vi "Actor Core.vi"(8 "error in":cluster{"状态":bool, "代码":i32, "源":string} caption="错误输入", 11 "客户端":refnum<class "客户端.lvclass"> caption="DNL_Beta") -> (0 "error out":cluster{"状态":bool, "代码":i32, "源":string} caption="错误输出", 3 "操作者输出":refnum<class "Actor.lvclass">)   [LabVIEW 2015, in "客户端操作者.lvlib" / "客户端.lvclass"]
doc: "Actor Core.vi包含操作者的主要消息处理循环。操作者通常位于该循环中，在各种消息到达时对消息进行处理。如Do.vi消息返回任何错误，该循环将停止运行，错误代码43将被作为“无错误停止”的标准信号发送给调用方。如需更改上述行为，可在子孙类的Handle Error.vi中对该部分逻辑进行重写。"
uses:
  <vilib>/ActorFramework/Actor/Actor.lvclass
panel:
  out "接收":string
  in  "发送按钮":bool
  in  "发送":string
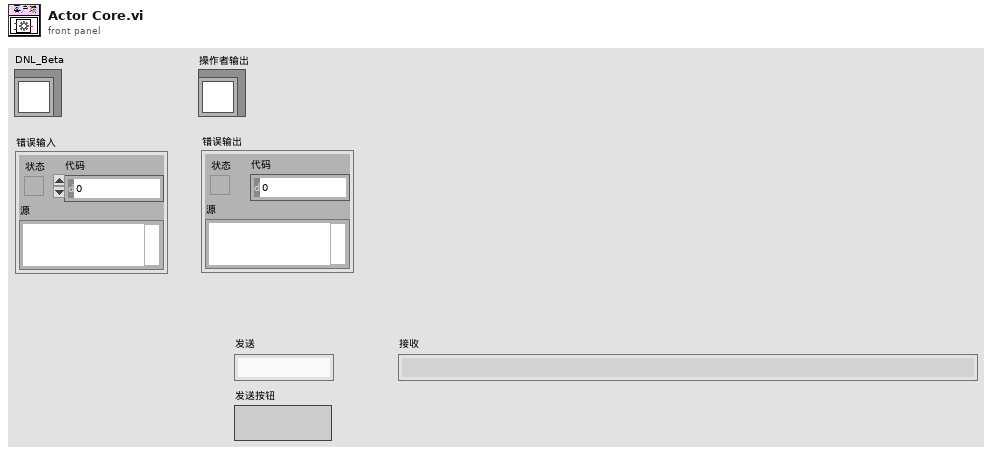
[diagram p1: front panel]
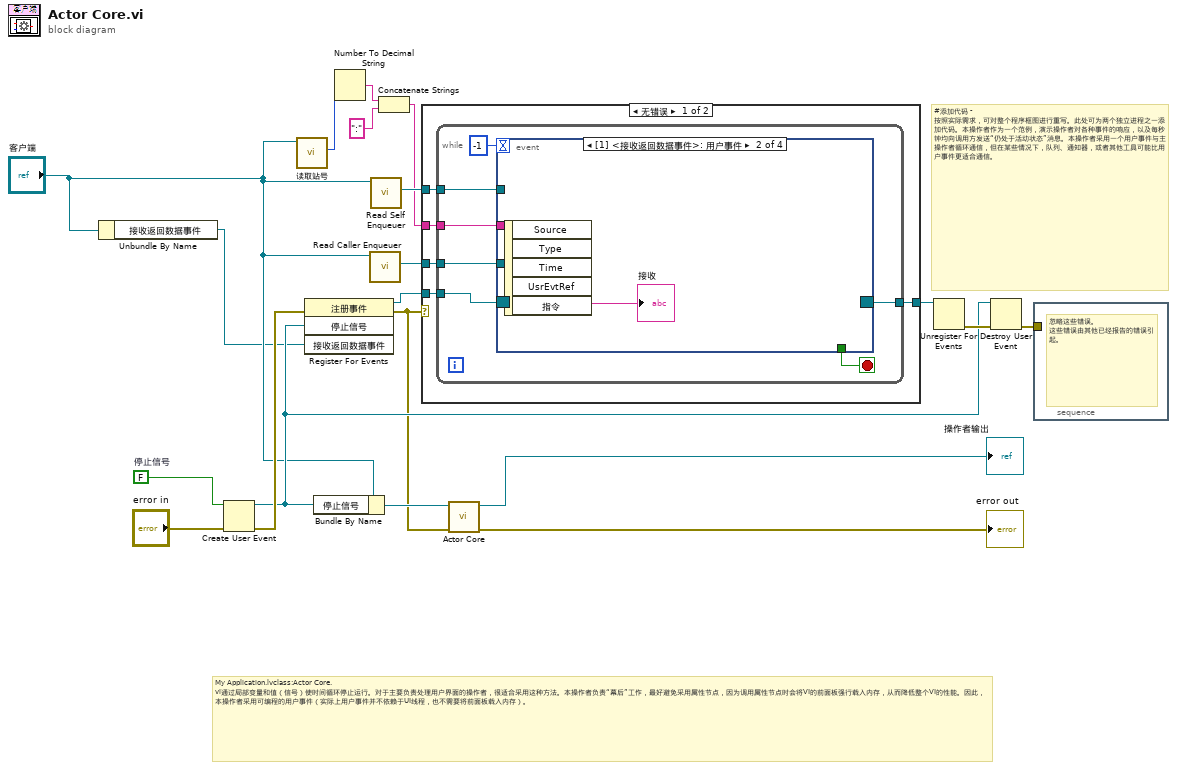
[diagram p0: block diagram]
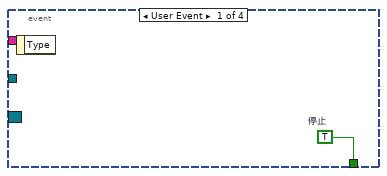
[diagram p2: hidden frame]
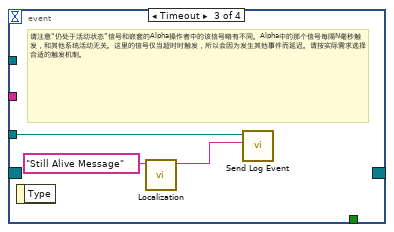
[diagram p3: hidden frame]
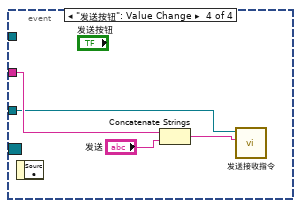
[diagram p4: hidden frame]
diagram:
  w16 = FALSE  # 停止信号
  # "My Application.lvclass:Actor Core.vi通过局部变量和值（信号）使时间循环停止运行。对于主要负责处理用户界面的操作者，很适合采用这种方法。本操作者负责“幕后”工作，最好避免采用属性节点，因为调用属性节点时会将VI的前面板强行载入内存，从而降低整个VI的性能。因此，本操作者采用可编程的用户事件（实际上用户事件并不依赖于UI线程，也不需要将前面板载入内存）。"
  # "#添加代码 - 按照实际需求，可对整个程序框图进行重写。此处可为两个独立进程之一添加代码。本操作者作为一个范例，演示操作者对各种事件的响应，以及每秒钟均向调用方发送“仍处于活动状态”消息。本操作者采用一个用户事件与主操作者循环通信，但在某些情况下，队列、通知器，或者其他工具可能比用户事件更适合通信。"
  n1 = Unbundle By Name("客户端") -> ("接收返回数据事件"=w3:refnum<user-event>)
  n2 = Create User Event(user event datatype=w16, error in="error in") -> (user event=w11:refnum<user-event>, error out=w15:errorcluster)
  n3 = call-dynamic "读取站号.vi"("客户端输入"="客户端") -> ("站号"=w8:u8)  [unwired: 8 in, 2 out]
  n4 = register-events(error in=w15, w11, w3) -> (reference out=w2:refnum<event-registration>, error out=w10:errorcluster)  [unwired: 1 in]
  n5 = Bundle By Name(cluster="客户端", "停止信号"=w11) -> (w13:refnum<class "客户端.lvclass">)
  n6 = Number To Decimal String(number=w8) -> (decimal integer string=w7:string)  [unwired: 1 in]
  n7 = call <vilib>:"Read Caller Enqueuer.vi"("Actor"="客户端") -> ("Caller Enqueuer"=w18:refnum<class "Message Enqueuer.lvclass">)  [unwired: 10 in]
  n8 = call <vilib>:"Read Self Enqueuer.vi"("Actor"="客户端") -> ("Self Enqueuer"=w19:refnum<class "Message Enqueuer.lvclass">)  [unwired: 10 in]
  n9 = Concatenate Strings(w7, ":") -> (w5:string)
  n10 = case shown="无错误" w10 {
    tunnel: w19 -> [w25 _]
    tunnel: w18 -> [w24 _]
    tunnel: w5 -> [w23 _]
    tunnel: w2 -> [w22 _]
    tunnel: [w21 _] -> w1
    frame No Error {
      n11 = while {
        tunnel: w25 -> [w31]
        tunnel: w24 -> [w30]
        tunnel: w23 -> [w29]
        tunnel: w22 -> [w28]
        tunnel: [w27] -> w21
        stop <- w32 stop-if-true
        n12 = event shown="[1] <接收返回数据事件>: 用户事件" {
          selector: w28 -> [_ _ _ _]
          dyn-events: [_ _ _ _] -> w27
          timeout: -1 -> [_ _ _ _]
          tunnel: [w33 _ _ _] -> w32
          tunnel: w31 -> [_ _ _ _]
          tunnel: w30 -> [_ _ w37 w39]
          tunnel: w29 -> [_ _ _ w41]
          event User Event {
            w33 = TRUE  # 停止
            n13 = event-data() -> ()  [unwired: 1 in, 1 out]
          }
          event User Event {
            n14 = event-data() -> ("指令"=→"接收":string)  [unwired: 1 in, 4 out]
          }
          event Timeout {
            # "请注意“仍处于活动状态”信号和嵌套的Alpha操作者中的该信号略有不同。Alpha中的那个信号每隔N毫秒触发，和其他系统活动无关。这里的信号仅当超时时触发，所以会因为发生其他事件而延迟。请按实际需求选择合适的触发机制。"
            n15 = event-data() -> ()  [unwired: 1 in, 1 out]
            n16 = call "Localization.vi"("未本地化"="Still Alive Message" ("Unlocalized")) -> ("本地化"=w35:string)  [unwired: 10 in]
            n17 = call "Send Log Event.vi"("事件文本"=w35, "消息待入队列"=w37) -> ()  [unwired: 9 in, 1 out]
          }
          event "发送按钮": Value Change {
            n18 = event-data() -> ()  [unwired: 1 in, 1 out]
            n19 = Concatenate Strings(w41, "发送") -> (w38:string)
            n20 = call "发送接收指令.vi"("接收指令"=w38, "Message Enqueuer"=w39) -> ()  [unwired: 8 in, 2 out]
          }
        }
      }
    }
    frame Error {
    }
  }
  n21 = call-parent "Actor Core.vi"("error in"=w10, "Actor in"=w13) -> ("error out"=→"error out":errorcluster, "Actor out"=→"操作者输出":refnum<class "Actor.lvclass">)  [unwired: 8 in]
  n22 = Unregister For Events(event registration refnum=w1) -> (error out=w12:errorcluster)  [unwired: 1 in]
  n23 = Destroy User Event(user event=w11, error in=w12) -> (error out=w9:errorcluster)
  n24 = stacked-sequence {
    tunnel: w9 -> [_]
    frame #0 {
      # "忽略这些错误。\n这些错误由其他已经报告的错误引起。"
    }
  }
